vi "TempMainProgramMarcoGonzalez.vi"() -> ()   [LabVIEW 2012]
panel:
  out "Numeric 2":dbl
  in  "Boolean":bool
  in  "Numeric":dbl
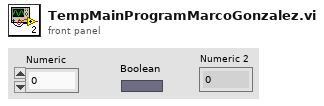
[diagram p1: front panel]
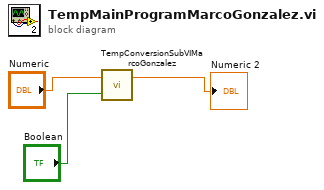
[diagram p0: block diagram]
diagram:
  n1 = call "TempConversionSubVIMarcoGonzalez.vi"("Boolean"="Boolean", "Temp"="Numeric") -> ("Converted Temp"=→"Numeric 2":dbl)  [unwired: 1 in]
